vi "Write Metadata.vi"(8 "error in (no error)":errorcluster, 10 "Metadata":refnum<class "Metadata.lvclass">[](array[class]), 11 "Add Metadata Msg in":refnum<class "Add Metadata Msg.lvclass">) -> (0 "error out":errorcluster, 3 "Add Metadata Msg out":refnum<class "Add Metadata Msg.lvclass">)   [LabVIEW 2020, in "Add Metadata Msg.lvclass"]
uses:
  Add Metadata Msg.lvclass
  Add Metadata Msg.lvclass/Add Metadata Msg.ctl
  NHMFL_Core/Libraries/File/Metadata/Metadata.lvclass
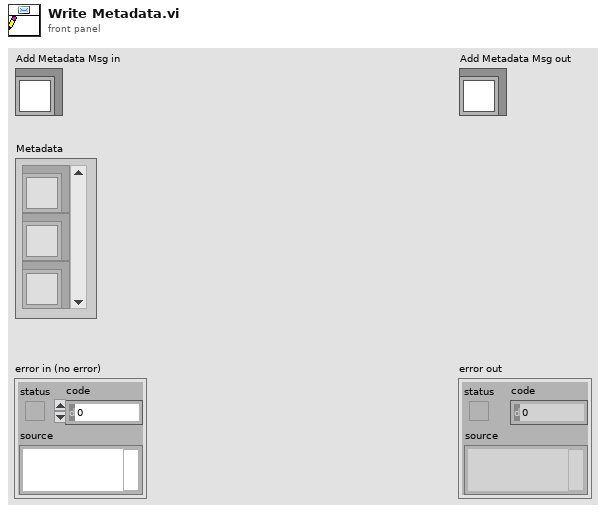
[diagram p1: front panel]
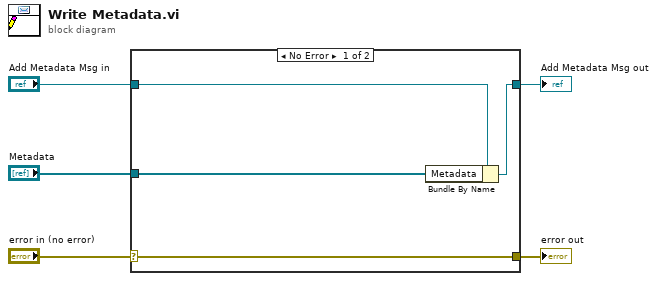
[diagram p0: block diagram]
diagram:
  n1 = case shown="No Error" "error in (no error)" {
    selector: "error in (no error)" -> [w9 w10]
    tunnel: [w9 w10] -> w4
    tunnel: [w7 w11] -> w2
    tunnel: "Add Metadata Msg in" -> [w8 w11]
    tunnel: "Metadata" -> [w6 _]
    frame No Error {
      n2 = Bundle By Name(cluster=w8, "Metadata"=w6) -> (w7:refnum<class "Add Metadata Msg.lvclass">)
    }
    frame Error {
    }
  }
  "error out" <- w4
  "Add Metadata Msg out" <- w2
